vi "Menu_global.vi"() -> ()   [LabVIEW 2017]
uses:
  Global 1.vi
panel:
  in  "Cowboy":bool
  in  "?":bool
  in  "Highball":bool
  in  "Jack & Coke":bool
  # "Cocktails Menu"
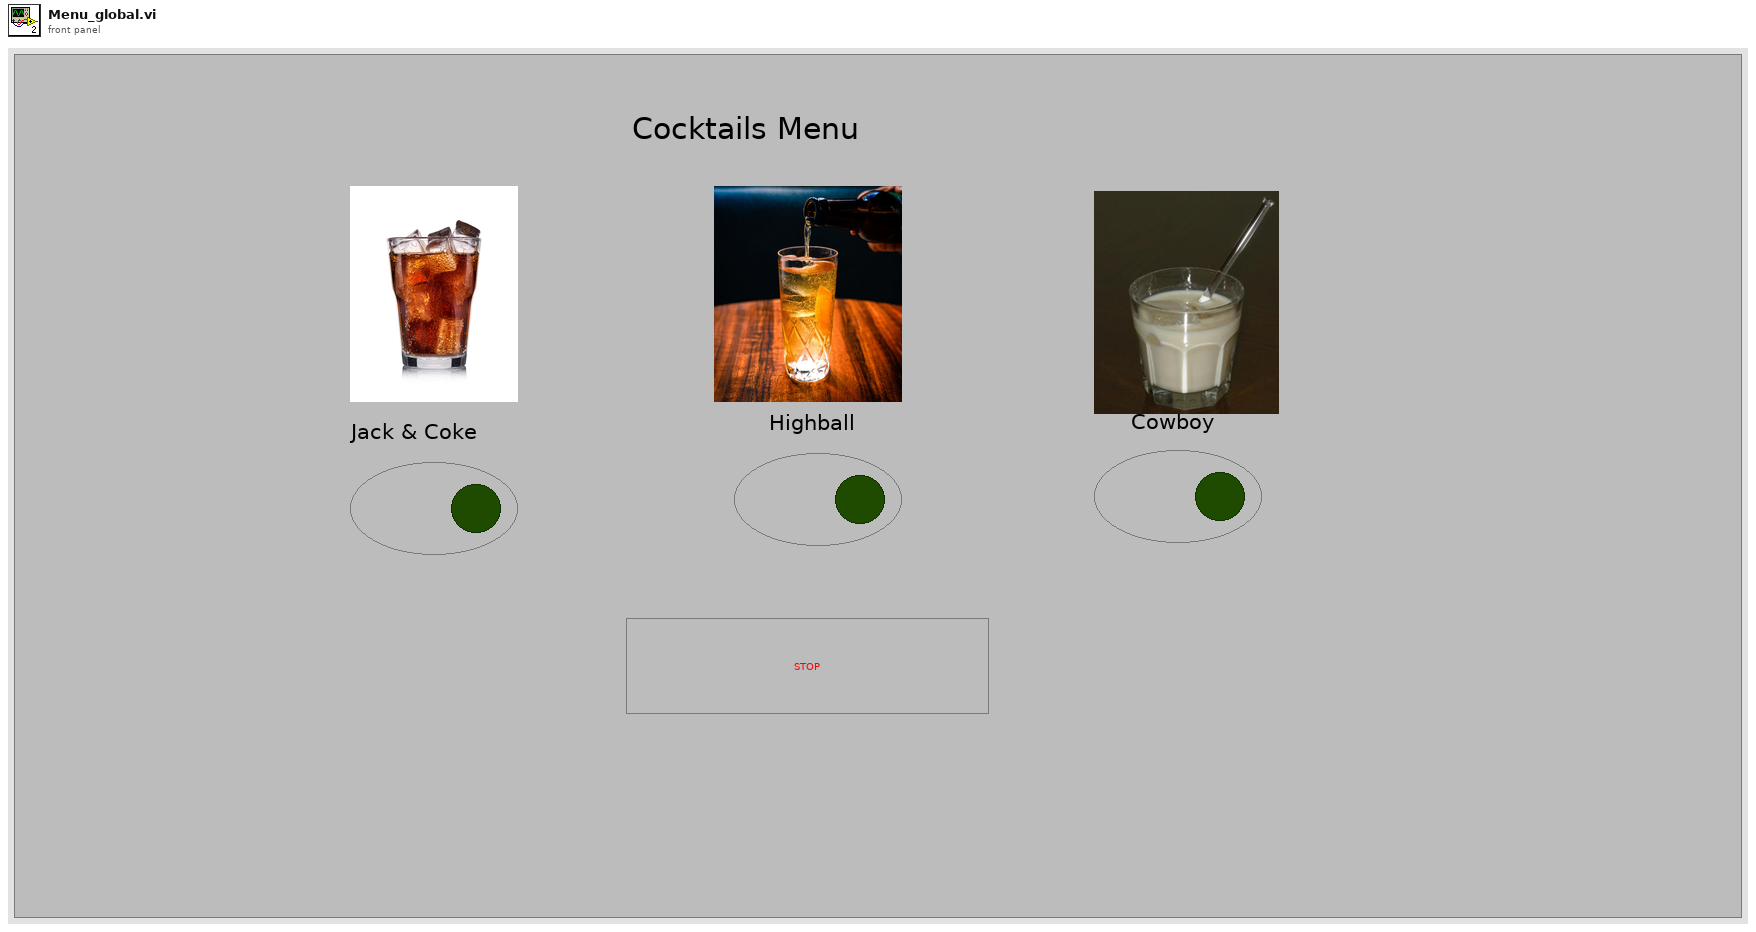
[diagram p1: front panel]
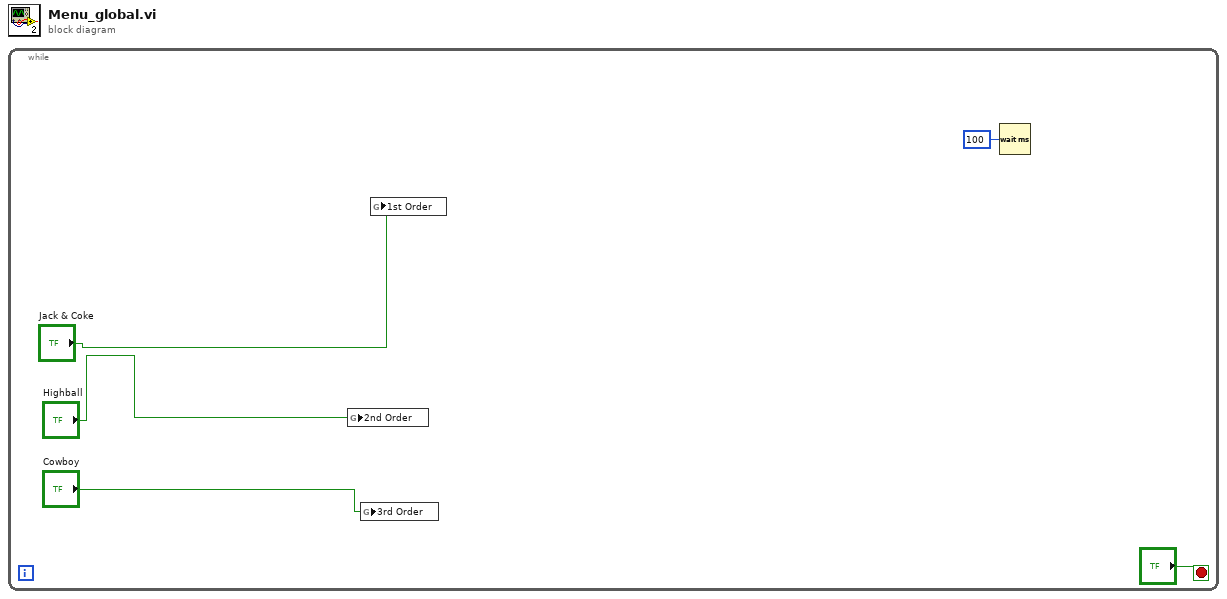
[diagram p0: block diagram]
diagram:
  n1 = while {
    stop <- "?" stop-if-true
    n2 = global write "Global 1.vi" "2nd Order"("Highball") -> ()
    n3 = global write "Global 1.vi" "3rd Order"("Cowboy") -> ()
    n4 = global write "Global 1.vi" "1st Order"("Jack & Coke") -> ()
    n5 = Wait (ms)(milliseconds to wait=u32 100) -> ()  [unwired: 1 out]
  }
